vi "AlliGator All ROIs IRF Analysis.vi"(8 "error in (no error)":errorcluster, 11 "AlliGator Internal Variables DVR":refnum<data-value>) -> (0 "error out":errorcluster, 1 "# IRFs defined":i32, 2 "Message":string, 3 "AlliGator Internal Variables DVR":refnum<data-value>)   [LabVIEW 2021, in "AlliGator Decay Analysis.lvlib" / "AlliGator IRF.lvlib"]
doc: "Extracts the decays from all ROIs and stores them as IRFs for subsequent NLSF analysis."
uses:
  AlliGator IRF.lvlib
  AlliGator Internal Variables v2.ctl
  <vilib>/vision/Image Controls.llb/IMAQ Image.ctl
  AlliGator Gate Image Set.ctl
  AlliGator FLI Dataset Type.ctl
  AlliGator Data Series Type.ctl
  AlliGator Dataset Channel.ctl
  AlliGator Gate Arithmetic.ctl
  AlliGator Displayed Image.ctl
  Image/Named ROI Description.ctl
  AlliGator Decay Metadata v3.ctl
  AlliGator Decay Background Subtraction Info.ctl
  AlliGator Baseline Subtraction Method.ctl
  Graphs/XY Graph/XY Graph Plot Shift Parameters.ctl
  Graphs/XY Graph/XY Graph Plot Shift Method.ctl
  AlliGator Decay Extrapolation Parameters.ctl
  Phasor/Calibration Phasor (m, phi).ctl
  Phasor/Phasor Reference Series.ctl
  Phasor/Phasor Calibration Map v2.ctl
  Phasor/Phasor (g, s).ctl
  AlliGator Raw Phasor Plot Data v4.ctl
  Phasor/Phasor Standard Deviation Options.ctl
  AlliGator Phasor Multi-Harmonic Data.ctl
  Phasor/Phasor Harmonic Data.ctl
  AlliGator Decay Fit Options & Parameters v2.ctl
  Fits/IRF(X)PSED/Decay Fit Options v2.ctl
  Fits/Decay Convolution/Decay Model.ctl
  Fits/Residual Type.ctl
  Fits/IRF(X)PSED/Fit Weights Type.ctl
  Fits/Non-linear Fitting Method v2.ctl
  Fits/Fit Calculation Method.ctl
  Fits/Non-linear Fitting Algorithm.ctl
  AlliGator Decay Fit Parameter Constraints 2.ctl
  Fits/IRF(X)PSED/Decay Fit Parameters In List.ctl
  Fits/IRF(X)PSED/MLE Baseline Offset Type.ctl
  AlliGator Decay Preprocessing Parameters.ctl
  Fits/IRF(X)PSED/Decay Fit Parameters & Derived Quantities List.ctl
  AlliGator Variables List.ctl
  Variant/Variant to Data/Variant to U16.vi
  <vilib>/Utility/error.llb/Error Cluster From Error Code.vi
  AlliGator Abort.vi
  <vilib>/ErrorRing/Error Ring.xnode
  AlliGator Globals, Variables & Constants.lvlib
  Image/Image.lvlib
  AlliGator Decay Processing.lvlib
  AlliGator Source Image.lvlib
  Strings/Strings.lvlib
  Time/Time.lvlib
  AlliGator Decay Preprocessing.lvlib
  Notebook/Notebook.lvlib
  Rich Text Box/Rich Text Box.lvlib
  GUI/GUI.lvlib
  Variant/Variant to Data/Variant to Data.lvlib
  Phasor/Phasor.lvlib
  AlliGator Files.lvlib
  AlliGator Internal Variables.lvlib
  AlliGator Phasor Graph.lvlib
  Graphs/XY Graph/XY Graph Add-Ons.lvlib
  AlliGator Phasor Plot.lvlib
  Fits/Fits.lvlib
  AlliGator Decay Fit.lvlib
  AlliGator Decay Fit Parameter Map.lvlib
  AlliGator Settings.lvlib
  AlliGator Dual-Channel Datasets.lvlib
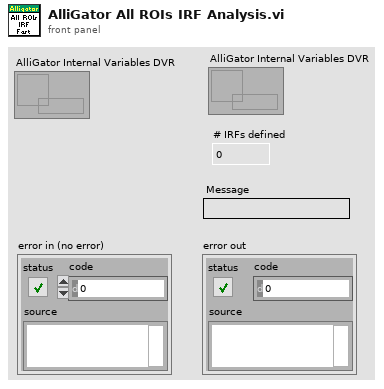
[diagram p1: front panel]
types:
  T1 = typedef "AlliGator Globals, Variables & Constants.lvlib/AlliGator Variables List.ctl" = enum16{"---- GUI ----", "Initialization Status", "State Indicators Refnum", "Original AlliGator Menu Items", "Current Action Loop State", "Script in progress", "Playback", "Loop Playback", "Search ROI Used", "Search ROI", "Decay Graph Max Legend Size", "Intensity Graph Max Legend Size", "Decay Statistics Graph Max Legend Size", "Phasor Graph Max Legend Size", "Phasor Ratio Graph Max Legend Size", "Lifetime Graph Max Legend Size", "---- Files ----", "Export Dataset Frames as Individual Files", "Show Batch Export Help Balloons", "Frames in Dataset", "ptu File Frame Start Indices", "Current Frame in Dataset", "Current Frame Timestamp", "------ Python Plugins ------", "Python Plugins Information", "Python Session", "Valid Python Session?", "---- Source Image ----", "Dataset Loaded", "Dataset Metadata", "Dataset Channel", "Dataset Data Description", "Background Dataset Metadata", "Background Dataset Channel", "Background Dataset Data Description", "Background File Subtraction", "Background File Path", "Background File Pile-up Correction", "Background File Pixel Well Capacity", "Background File Scaling Factor", "Source Image ROIs", "Current Source Image ROI", "Source Image ROI Event Refnum", "X_Source Image Display Range", "X_Source Image Palette Information", "Source Image Palette List", "Source Image Scale", "Current Dataset Load Settings", "Source Image:ROI Overlay Color", "---- Image Profile Window ----", "Image Profile:Overlay ROI in Source Image", "Image Profile Window Event Refnum", "Image Profile:IntensityType", "Image Profile:Intensity Average Type", "Image Profile:Intensity-weighted SDV", "Image Profile:Box Profile Type", "Image Profile Window Open", "Image Profile:Plotted Fit Parameter", "X_Type of Displayed Image", "X_Time Gate Slider", "Dataset Path", "Source Image Overlay to Erase", "Is Displayed Image Accumulated", "White Light Image Modified", "Mask Image Modified", "Macrotime Gate Separation", "------ Phasor Graph -------", "Phasor Graph:Show Line", "---- Phasor Plot ---", "Phasor Plot Parameters Changed", "FLI Dataset Modified since last Phasor Plot Calculation", "Phasor Harmonics Data", "Selected Phasor Harmonics", "Phasor Harmonic Manager Event Refnum", "Phasor Plot ROIs", "Current Phasor Plot ROI", "Phasor Plot ROI Event Refnum", "Phasor Plot Image Reference Points", "Phasor Plot Computed", "Phasor Plot Palette Information", "Phasor Plot Palette List", "Phasor Ratio Palette Information", "Phasor Ratio Palette List", "Phasor Image Scale", "Phasor Plot Image Overlay to Erase", "Phasor Plot Image Elements to Update", "Current Phasor Plot Calculation Parameters", "Current Phasor Calibration Options", "Reset Cumulated Phasor Plot", "Phasor Ratio Reference 1", "Phasor Ratio Lifetime Reference 1", "Phasor Ratio Reference 1 Frequency", "Phasor Ratio Reference 2", "Phasor Ratio Lifetime Reference 2", "Phasor Ratio Reference 2 Frequency", "---- Decay Analysis ----", "Number of Selected Decays to Fit", "LS Fit Results", "LAR Fit Results", "BS Fit Results", "Last Decay Max - Min", "Best Fit Parameters", "Best Fit Parameter Names", "Actual Size X", "Actual Size Y", "Binning X", "Binning Y", "Actual # Gates", "Dataset Number", "Gates to...", "Gates Skipped", "Gates to keep", "Gate Step", "Gate Separation", "Reversed Gates", "Pile-up Correction", "Pixel Well Capacity", "Background Subtracted", "Background Subtraction Method", "Background Definition Range", "Background File (deprecated)", "Number of Dataset Accumulated", "Array of Accumulated Dataset Paths", "Do Averaged Datasets", "Destination File Path", "Process Plot Target", "Use 1/D as Phasor Frequency", "---- Decay Fit Parameter Map -----", "Decay Fit Parameter Map Palette Information", "Decay Fit Parameter Map Palette List", "Local Decay Graph Window Event Refnum", "------- Local Decay Window ---------", "Use normalized IRF for convolution", "----- Miscellaneous ----", "Skippable Dialog Windows Status"}
  T2 = typedef "IMAQ Image.ctl" = refnum<image>
  T3 = typedef "Image.lvlib/Named ROI Description.ctl" = cluster{"ROI Descriptor":T4, "ROI Name":string, "Overlay Color":u32}
  T4 = typedef "ROI Descriptor" = cluster{"Global Rectangle":i32[], "Contours":cluster{"ID":enum32{"External", "Internal"}, "Type":u32, "Coordinates":i32[]}[]}
  T5 = typedef "AlliGator Internal Variables.lvlib/AlliGator Internal Variables v2.ctl" = cluster{"Displayed Image":T2, "White Light Image":T2, "Mask Image":T2, "ROI Mask Image":T2, "Current Dataset Images 1":T6, "Background Dataset Images 1":T6, "Current Dataset Images 2":T6, "Background Dataset Images 2":T6, "Current Dataset Arithmetic Images":T6, "Accumulated Dataset Images 1":T6, "Accumulated Dataset Images 2":T6, "Accumulated Dataset Arithmetic Images":T6, "Phasor Plot Image":T2, "Decay Fit Parameter Map Image":T2, "Single Data Point Path":path, "White Light Image Path":path, "Mask Image Path":path, "Time-Series Folder":path, "[Time-Series Paths]":path[], "Current Dataset":i32, "Single Dataset Type":T7, "Current Folder":string, "AlliGator Data Series Type":T8, "# Datasets":i32, "Dual-Channel Dataset":bool, "Selected Channel Name":string, "Dataset Channel":T9, "Channel Arithmetic":T10, "Dual-Channel Background Dataset":bool, "Background Channel":T9, "Dual-Channel Accumulated Dataset":bool, "Start Time":dbl, "[Time-Series Timestamps]":dbl[], "[Intensity Corrections]":dbl[], "Time Series Script":bool, "Type of Displayed Image":T11, "Gate Image Slide":u16, "# Gates":i32, "ROIs":T3[], "ROI Decay":cluster{"t Array":dbl[], "I Array":dbl[]}, "Valid Decay":bool, "Decay  Metadata":T12, "Reference Decay Plot Name":string, "Reference Decay":cluster{"t Array":dbl[], "I Array":dbl[]}, "Decay Shift Plot":cluster{"Time Stamps":dbl[], "Decay Shifts":dbl[]}, "[Decays Max Values]":sgl[], "[Decays Min Values]":sgl[], "Calibration Phasor":T18, "Calibration Phasor Series":T19, "Phasor Calibration Map":T20, "Calibration Map MD5 Digest":string, "Last Raw Phasor":T21, "Last Calibrated Phasor":T21, "Last Calibrated Phasor SDV":T21, "Phasor Graph:Phasor Plot":cluster{"g Array":dbl[], "s Array":dbl[]}, "Phasor Graph:Phasor SDV Plot":cluster{"g Array":dbl[], "s Array":dbl[]}, "[Phasor Graph:Raw Phasor Plots]":T22[], "Phasor Plot locked to Ref 1":i32, "[Phasor Plot(s) locked to Ref 1]":i32[], "[Phasor Plot(s) locked to Ref 2]":i32[], "[Pixel Phasors]":T21[], "[[Sum Image]]":dbl[][], "[[CSG Phasors]]":csg[][], "[[Valid Pixel?]]":bool[][], "I/m/phi Dataset":cluster{"I/m/phi Dataset?":bool, "Base Frequency":dbl[unit], "Harmonic Orders":u8[]}, "Multi Phasor Plot Data":T24, "Decay Fit Options & Parameters":T26, "Fit Options: Decay Preprocessing Parameters":T37, "Fit Options: Reference Decay":cluster{"t Array":dbl[], "I Array":dbl[]}, "Is Full Image Parameters Map":bool, "Is Single-Pixels Parameters Map":bool, "NLSF Parameters Map X Resolution":i32, "NLSF Parameters Map Y Resolution":i32, "[Single Decay Fit Parameters]":dbl[], "Fit Model":T28, "[[Multiple Decays Fit Parameters]]":dbl[][], "[[Multiple Decays Fit Parameter SDVs]]":dbl[][], "[[IRFs]]":dbl[][], "IRF Array Time Axis":dbl[], "Decay Array Time Axis":dbl[], "[Decay Fit Parameter Names]":T38[], "[[Phasor Ratios]]":dbl[][], "[[Average Lifetimes]]":dbl[][], "Amplitude Weighted Average Lifetime":bool, "[Decay Sum]":dbl[], "[[User-defined Quantities]]":dbl[][], "User-defined Quantity":string}
  T6 = typedef "AlliGator Files.lvlib/AlliGator Gate Image Set.ctl" = cluster{"SGL Image Max":T2, "SGL Image Sum":T2, "SGL Gate Images":T2[], "SGL Image Min":T2}
  T7 = typedef "AlliGator Files.lvlib/AlliGator FLI Dataset Type.ctl" = enum16{"HDF5 FLI Dataset", "Gate Image Folder", ".sdt FLI Dataset (Becker & Hickl)", ".ptu FLI Dataset (PicoQuant)", "SS1 FLI Dataset", "SS2 FLI Dataset", "I/m/phi Dataset", ".bin FLI Dataset (PicoQuant Binned)", ".bin FLI Dataset (Piccolo Binned)"}
  T8 = typedef "AlliGator Files.lvlib/AlliGator Data Series Type.ctl" = enum16{"Not a Supported Series", "Gate Images Folder Series", "SwissSPAD 2 Dataset Series", "B&H FLI Dataset Series", "PicoQuant PTU FLI Dataset Series", "PicoQuant BIN FLI Dataset Series", "Piccolo hist BIN FLI Dataset Series", "HDF5 FLI Dataset Series"}
  T9 = typedef "AlliGator Dual-Channel Datasets.lvlib/AlliGator Dataset Channel.ctl" = enum16{"G2", "INT"}
  T10 = typedef "AlliGator Settings.lvlib/AlliGator Gate Arithmetic.ctl" = enum16{"None", "INT-G2", "G2/INT*<INT>", "(1 - G2/INT)*<INT>"}
  T11 = typedef "AlliGator Source Image.lvlib/AlliGator Displayed Image.ctl" = enum16{"Single Gate", "Sum of All Gates", "Max of All Gates", "Min of All Gates", "-", "White Ligth Image", "Mask Image"}
  T12 = typedef "AlliGator Phasor Graph.lvlib/AlliGator Decay Metadata v3.ctl" = cluster{"ROI Descriptor":T4, "ROI Center":cluster{"X":i32, "Y":i32}, "Decay Background Subtraction Info":T13, "Decay Reverted":bool, "Decay Smoothened":bool, "Decay Straightened":bool, "Fitted Tau (Decay Straightening)":dbl, "Decay Shift Parameters":T15, "Decay Shifted":bool, "Decay Extrapolated":bool, "Decay Extrapolation Parameters":T17, "Decay Normalized":bool, "Fold Decay":bool, "# Folds":u32}
  T13 = typedef "AlliGator Decay Analysis.lvlib/AlliGator Decay Preprocessing.lvlib/AlliGator Decay Background Subtraction Info.ctl" = cluster{"Laser Period":dbl[unit], "Gate Duration":dbl[unit], "Baseline Subtraction Method":T14, "Background Definition Range":cluster{"Min Gate":dbl[unit], "Max Gate":dbl[unit]}, "Total Intensity w/o Bkgd Subtraction":dbl, "Bkgd-subtracted Intensity (exp)":dbl, "# Data Points":i32, "Background/Gate":dbl, "Fitted Lifetime":dbl[unit], "Bkgd-subtracted Intensity (theo)":dbl}
  T14 = typedef "AlliGator Decay Analysis.lvlib/AlliGator Decay Preprocessing.lvlib/AlliGator Baseline Subtraction Method.ctl" = enum16{"Mean", "Min", "Square Gated Single-Exponential", "File", "Constant"}
  T15 = typedef "XY Graph Add-Ons.lvlib/XY Graph Plot Shift Parameters.ctl" = cluster{"Type":T16, "Shift":dbl[unit], "Threshold":dbl, "Rotate":bool}
  T16 = typedef "XY Graph Add-Ons.lvlib/XY Graph Plot Shift Method.ctl" = enum16{"Default", "CFD", "Threshold", "Cross-Correlation"}
  T17 = typedef "AlliGator Decay Analysis.lvlib/AlliGator Decay Preprocessing.lvlib/AlliGator Decay Extrapolation Parameters.ctl" = cluster{"Additional Points":u32, "Head Fraction":dbl, "Fitted Tau":dbl, "Use Periodicity":bool, "Use Cursors":bool, "Tail Fraction":dbl}
  T18 = typedef "Phasor.lvlib/Calibration Phasor (m, phi).ctl" = cluster{"m":dbl, "phi":dbl, "Phasor Frequency":dbl[unit], "Reference Lifetime":dbl[unit]}
  T19 = typedef "Phasor.lvlib/Phasor Reference Series.ctl" = cluster{"m Array":dbl[], "phi Array":dbl[], "Phasor Frequency":dbl[unit], "Calibration Lifetime":dbl[unit]}
  T20 = typedef "Phasor.lvlib/Phasor Calibration Map v2.ctl" = cluster{"Phasor Frequency":dbl[unit], "Calibration Lifetime":dbl[unit], "ROI Centers":cluster{"X":i32, "Y":i32}[], "ROI Descriptors":T4[], "Map Resolution X":i32, "Map Resolution Y":i32, "z Array":cdb[]}
  T21 = typedef "Phasor.lvlib/Phasor (g, s).ctl" = cluster{"g":dbl, "s":dbl}
  T22 = typedef "AlliGator Phasor Graph.lvlib/AlliGator Raw Phasor Plot Data v4.ctl" = cluster{"Phasor Plot Name":string, "Raw Phasor Plot":T21[], "Phasor Frequency":dbl[unit], "[Decay Metadata]":T12[], "Raw Phasor Plot SDV":T21[], "Phasor SDV Options":T23, "[Calibration Phasor]":T18[]}
  T23 = typedef "Phasor.lvlib/Phasor Standard Deviation Options.ctl" = cluster{"Compute Estimated SDV":bool, "# Replicas":u32, "Use Estimated Average Phasor":bool}
  T24 = typedef "AlliGator Phasor Plot.lvlib/AlliGator Phasor Multi-Harmonic Data.ctl" = cluster{"Base Frequency":dbl[unit], "# Harmonics":u8, "Harmonic Orders":u8[], "Phasor Plot Settings Checksum":u64, "Phasor Harmonic Data Array":T25[]}
  T25 = typedef "Phasor.lvlib/Phasor Harmonic Data.ctl" = cluster{"Phasor Harmonic Name":string, "Phasor Plot Settings Checksum":u64, "Phasor Frequency":dbl[unit], "Base Frequency":dbl[unit], "Harmonic Order":u8, "Phasor Plot Parameters":string, "Phasor Array [[CSG]]":csg[][], "Dataset File Path":path}
  T26 = typedef "AlliGator Decay Fit Parameter Map.lvlib/AlliGator Decay Fit Options & Parameters v2.ctl" = cluster{"SYNC Period":dbl[unit], "Fit Options":T27, "Fit Parameter Constraints":T34[], "MLE Baseline Offset":dbl, "MLE Baseline Offset Type":T36}
  T27 = typedef "Fits.lvlib/Decay Fit Options v2.ctl" = cluster{"Show Fit Residuals":bool, "Fit Model":T28, "Residual Type":T29, "Max Decay Percentile":dbl, "Min Decay Percentile":dbl, "Show Full Decay":bool, "Weights":T30, "Fitting Method":T31, "Compute Parameter Uncertainties":bool, "Periodic Boundaries":bool, "Model Calculation":T32, "Period":dbl[unit], "Termination Criteria":cluster{"Max Iterations":i32, "Max Function Calls":i32, "Max Time":dbl[unit], "Function Tolerance":dbl, "Parameter Tolerance":dbl, "Gradient Tolerance":dbl, "Min Lambda":dbl, "Max Lambda":dbl, "Initial Tick Count":u32}, "Offset Resolution":dbl[unit], "Use Local IRF":bool, "Fitting Algorithm":T33}
  T28 = typedef "Fits.lvlib/Decay Model.ctl" = enum16{"1-Exponential", "2-Exponentials"}
  T29 = typedef "Fits.lvlib/Residual Type.ctl" = enum16{"Standard", "Normalized", "Reduced"}
  T30 = typedef "Fits.lvlib/Fit Weights Type.ctl" = enum16{"Unweighted", "1/Variance", "Best of All"}
  T31 = typedef "Fits.lvlib/Non-linear Fitting Method v2.ctl" = enum16{"Least Square", "Least Absolute Residual", "Bisquare", "MLE", "-", "Best of All"}
  T32 = typedef "Fits.lvlib/Fit Calculation Method.ctl" = enum16{"Simulation", "Convolution", "Integration"}
  T33 = typedef "Fits.lvlib/Non-linear Fitting Algorithm.ctl" = enum16{"Levenberg-Marquardt", "Trust-Region Dogleg"}
  T34 = typedef "AlliGator Decay Analysis.lvlib/AlliGator Decay Fit.lvlib/AlliGator Decay Fit Parameter Constraints 2.ctl" = cluster{"Fit Parameter":T35, "Min Value":dbl, "Max Value":dbl, "Global":bool, "Used":bool}
  T35 = typedef "Fits.lvlib/Decay Fit Parameters In List.ctl" = enum16{"Offset", "Baseline", "A_1", "tau_1", "A_2", "tau_2"}
  T36 = typedef "Fits.lvlib/MLE Baseline Offset Type.ctl" = enum32{"Absolute", "Percentage"}
  T37 = typedef "AlliGator Decay Analysis.lvlib/AlliGator Decay Preprocessing.lvlib/AlliGator Decay Preprocessing Parameters.ctl" = cluster{"Background Subtraction":bool, "Straighten Decay":bool, "Reverse Gates":bool, "1-Normalized Decay":bool, "Smoothen Decay":bool, "Smoothing Parameter":dbl, "Shift Decay":bool, "Decay Shift Parameters":T15, "Extrapolate Decay":bool, "Additional Points":u32, "Head Fraction":dbl, "Pixel-Normalize Decay":bool, "Use Periodicity":bool, "Use Cursors":bool, "Tail Fraction":dbl, "Use Decay Pre-Processing":bool, "Fold Decay":bool, "# Folds":u32, "[0-1]-Normalized Decay":bool}
  T38 = typedef "Fits.lvlib/Decay Fit Parameters & Derived Quantities List.ctl" = enum16{"Offset", "Baseline", "A_1", "tau_1", "A_2", "tau_2", "<tau>_a", "f1_a", "f2_a", "<tau>_i", "f1_i", "f2_i", "-", "R^2", "Chi^2"}
  T39 = typedef "AlliGator Settings.lvlib/AlliGator Pixel Counts Constraints.ctl" = cluster{"High Count Pixels Rejection Options":T40, "Low Count Pixels Rejection Options":T41}
  T40 = typedef "AlliGator Settings.lvlib/AlliGator High Count Pixels Rejection Options.ctl" = cluster{"Background High Threshold Factor":dbl, "Fixed High Background Threshold":dbl, "Reject High Count Pixels":bool, "High Percentile":dbl}
  T41 = typedef "AlliGator Settings.lvlib/AlliGator Low Count Pixels Rejection Options.ctl" = cluster{"Background Low Threshold Factor":dbl, "Fixed Low Background Threshold":dbl, "Reject Low Count Pixels":bool, "Low Percentile":dbl}
  T42 = cluster{"Decay Peak Constraint":bool, "Min":dbl, "Max":dbl}
  T43 = typedef "Rich Text Box.lvlib/Text Formatting.ctl" = cluster{"Font":string, "Text Color":T44, "Text Background Color":T44, "Text Style":enum16{"Regular", "Bold", "Italic", "Underline", "Strikeout"}, "Font Size (Points)":dbl, "Text Alignment":i32}
  T44 = typedef "Rich Text Box.lvlib/Text Colors.ctl" = enum16{"Unchanged", "Black", "Blue", "Brown", "Gray", "Green", "Orange", "Pink", "Red", "White"}
  T45 = cluster{"t Axis":dbl[], "ROI Intensity Array":dbl[]}
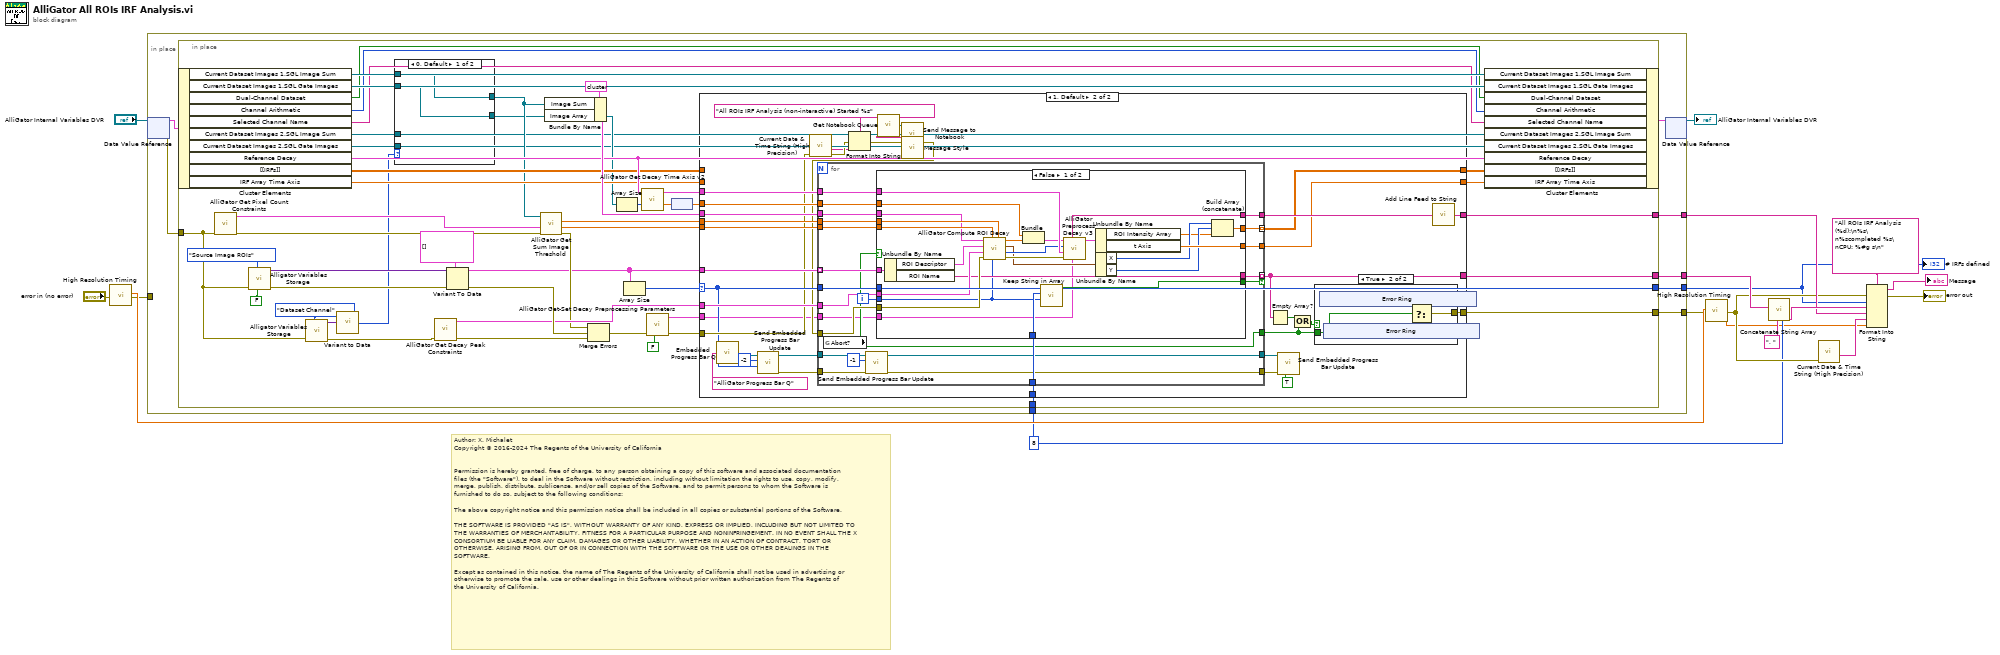
[diagram p0: block diagram]
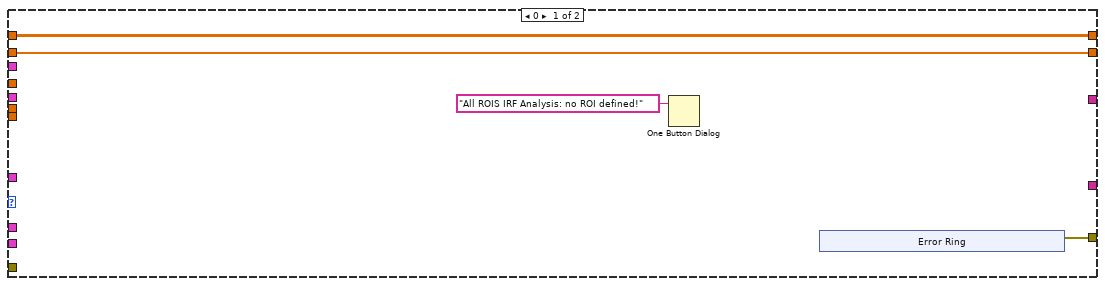
[diagram p3: hidden frame]
diagram:
  w6 = 8 ("Max Number of Elements (None: -1)")
  # "Author: X. Michalet\nCopyright © 2016-2024 The Regents of the University of California\n \n\nPermission is hereby granted, free of charge, to any person obtaining a copy of this software and associated documentation files (the \"Software\"), to deal in the Software without restriction, including without limitation the rights to use, copy, modify, merge, publish, distribute, sublicense, and/or sell copies of the Software, and to permit persons to whom the Software is furnished to do so, subject to the following conditions:\n\nThe above copyright notice and this permission notice shall be included in all copies or substantial portions of the Software.\n\nTHE SOFTWARE IS PROVIDED \"AS IS\", WITHOUT WARRANTY OF ANY KIND, EXPRESS OR IMPLIED, INCLUDING BUT NOT LIMITED TO THE WARRANTIES OF MERCHANTABILITY, FITNESS FOR A PARTICULAR PURPOSE AND NONINFRINGEMENT. IN NO EVENT SHALL THE X CONSORTIUM BE LIABLE FOR ANY CLAIM, DAMAGES OR OTHER LIABILITY, WHETHER IN AN ACTION OF CONTRACT, TORT OR OTHERWISE, ARISING FROM, OUT OF OR IN CONNECTION WITH THE SOFTWARE OR THE USE OR OTHER DEALINGS IN THE SOFTWARE.\n\nExcept as contained in this notice, the name of The Regents of the University of California shall not be used in advertising or otherwise to promote the sale, use or other dealings in this Software without prior written authorization from The Regents of the University of California."
  n1 = call "High Resolution Timing.vi"("Error In"="error in (no error)") -> ("elapsed (relative) seconds"=w13:dbl, "Error Out"=w10:errorcluster)  [unwired: 16 in, 1 out]
  n2 = in-place {
    in-place-border: [w24] -> w7
    in-place-border: [w23] -> w11
    in-place-border: w10 -> [_]
    in-place-border: [w21] -> w9
    in-place-border: [w20] -> w5
    in-place-border: w6 -> [w19]
    n3 = in-place-dvr #1("AlliGator Internal Variables DVR") -> (w26:T5, w22:errorcluster)
    n4 = in-place {
      in-place-border: w22 -> [w29]
      in-place-border: [w57] -> w24
      in-place-border: [w48] -> w23
      in-place-border: [w56] -> w21
      in-place-border: [w50] -> w20
      in-place-border: w19 -> [w49]
      n5 = in-place-cluster #2(w26) -> ("Current Dataset Images 1.SGL Image Sum"=w38:T2, "Current Dataset Images 1.SGL Gate Images"=w37:T2[], "Dual-Channel Dataset"=w32:bool, "Channel Arithmetic"=w33:T10, "Selected Channel Name"=w34:string, "Current Dataset Images 2.SGL Image Sum"=w36:T2, "Current Dataset Images 2.SGL Gate Images"=w35:T2[], "Reference Decay"=w58:cluster{"t Array":dbl[], "I Array":dbl[]}, "[[IRFs]]"=w45:dbl[][], "IRF Array Time Axis"=w44:dbl[])
      n6 = call "AlliGator Get Pixel Count Constraints.vi"("error in (no error)"=w29) -> ("error out"=w67:errorcluster, "Pixel Count Constraints"=w68:T39)  [unwired: 9 in]
      n7 = call "Alligator Variables Storage.vi"("Get(F)/Set"=FALSE, "AlliGator Variable"=AlliGator_Variables_List."Source Image ROIs" ("Alligator Variable"), "Error In"=w29) -> ("Error Out"=w71:errorcluster, "Data out"=w72:variant)  [unwired: 6 in, 1 out]
      n8 = call "Alligator Variables Storage.vi"("AlliGator Variable"=AlliGator_Variables_List."Dataset Channel" ("Alligator Variable"), "Error In"=w29) -> ("Error Out"=w28:errorcluster, "Data out"=w30:variant)  [unwired: 7 in, 1 out]
      n9 = call-poly "Variant to Data.vi"("Variant"=w30) -> ("U16 Value"=w27:u16)  [unwired: 8 in]
      n10 = case shown="0, Default" w27 {
        tunnel: [w75 w77] -> w40
        tunnel: w36 -> [_ w77]
        tunnel: [w74 w76] -> w39
        tunnel: w35 -> [_ w76]
        tunnel: w38 -> [w75 _]
        tunnel: w37 -> [w74 _]
        frame 0, Default {
        }
        frame 1 {
        }
      }
      n11 = call "AlliGator Get Decay Peak Constraints.vi"("error in (no error)"=w28) -> ("Error Out"=w63:errorcluster, "Decay Peak Constraints"=w62:T42)  [unwired: 9 in]
      n12 = Variant To Data(error in=w71, type=T3[] [] ("Stored ROIs in"), Variant=w72) -> (data=w51:T3[], error out=w66:errorcluster)
      n13 = call "AlliGator Get Sum Image Threshold.vi"("error in (no error)"=w67, "Pixel Counts Constraints"=w68, "Image in"=w40) -> ("error out"=w55:errorcluster, "Pixel Threshold Low"=w64:sgl, "Pixel Threshold High"=w65:sgl)  [unwired: 2 in, 4 out]
      n14 = Bundle By Name(cluster=cluster{"Image Sum":T2, "Image Array":T2[]} {"Image Sum"=refnum, "Image Array"=[]} ("Images"), "Image Sum"=w40, "Image Array"=w39) -> (w61:cluster{"Image Sum":T2, "Image Array":T2[]})
      n15 = Merge Errors(w55, w66, w63) -> (w47:errorcluster)
      n16 = Array Size(array=w39) -> (size(s)=w60:i32)
      n17 = Array Size(array=w51) -> (size(s)=w50:i32)
      n18 = call "AlliGator Get Decay Time Axis v2.vi"("Number of Gates"=w60) -> ("t Array"=w59:dbl[unit][])  [unwired: 14 in]
      n19 = call "AlliGator Get-Set Decay Preprocessing Parameters.vi"("Get (F)/Set"=FALSE, "Error In"=w47) -> ("Error Out"=w46:errorcluster, "Decay Preprocessing Parameters out"=w42:T37)  [unwired: 8 in]
      n20 = node(w59) -> (w54:dbl[])
      n21 = case shown="1, Default" w50 {
        selector: w50 -> [_ w92]
        tunnel: w65 -> [_ w121]
        tunnel: w64 -> [_ w120]
        tunnel: w62 -> [_ w119]
        tunnel: w61 -> [_ w118]
        tunnel: w58 -> [_ w117]
        tunnel: [w79 w116] -> w57
        tunnel: [_ w112] -> w56
        tunnel: w54 -> [_ w111]
        tunnel: [w80 w109] -> w53
        tunnel: [w81 w108] -> w52
        tunnel: w51 -> [_ w107]
        tunnel: w49 -> [_ w106]
        tunnel: [_ w105] -> w48
        tunnel: w46 -> [_ w98]
        tunnel: w45 -> [w81 _]
        tunnel: w44 -> [w80 _]
        tunnel: w42 -> [_ w87]
        frame 0 {
          n22 = One Button Dialog(message="All ROIS IRF Analysis: no ROI defined!") -> ()  [unwired: 1 in, 1 out]
          n23 = xnode "Error Ring"() -> ("error out"=w79:errorcluster)
        }
        frame 1, Default {
          n24 = call "Embedded Progress Bar Q.vi"("Progress Bar Queue Name"="AlliGator Progress Bar Q") -> ("Progress Bar Queue"=w95:refnum<queue>)  [unwired: 6 in]
          n25 = call "Send Embedded Progress Bar Update.vi"("Max Iterations N"=w92, "Current Iteration i (i or -1: standard or || iteration; 0 or -2: first standard or || iteration)"=-2 ("Current Iteration i (-1: || iteration, -2: first || iteration)"), "Progress Bar Queue in"=w95) -> ("Error Out"=w91:errorcluster, "Progress Bar Queue out"=w93:refnum<queue>)  [unwired: 7 in]
          n26 = call "Current Date & Time String (High Precision).vi"("Error In"=w98) -> ("Error Out"=w100:errorcluster, "on <Date> at <Time>"=w86:string)  [unwired: 7 in, 2 out]
          n27 = Format Into String(format string="All ROIs IRF Analysis (non-interactive) Started %s", error in=w100, w86) -> (resulting string=w97:string, error out=w102:errorcluster)  [unwired: 1 in]
          n28 = call "Get Notebook Queue.vi"() -> ("Notebook Queue"=w101:refnum<queue>)  [unwired: 9 in]
          n29 = call "Message Style.vi"() -> ("Message Formatting"=w103:T43)
          n30 = call "Send Message to Notebook.vi"("Text Formatting"=w103, "Error In"=w102, "Message"=w97, "Notebook Queue"=w101) -> ("Error Out"=w99:errorcluster)  [unwired: 4 in, 1 out]
          n31 = for {
            tunnel: w107 -> [w156] mode=indexing
            tunnel: w121 -> [w155]
            tunnel: w120 -> [w154]
            tunnel: w118 -> [w153]
            tunnel: w119 -> [w152]
            tunnel: [w140] -> w110
            tunnel: w111 -> [w148]
            tunnel: w117 -> [w149]
            tunnel: [w150] -> w105 mode=indexing if=w144
            tunnel: w99 -> [w151]
            tunnel: [w147] -> w113
            tunnel: [w146] -> w109
            tunnel: [w145] -> w108 mode=indexing
            tunnel: w92 -> [w142]
            tunnel: w106 -> [w141]
            tunnel: w93 -> [w138]
            tunnel: w91 -> [w137]
            tunnel: [w136] -> w90
            tunnel: [w135] -> w89
            tunnel: w87 -> [w134]
            i -> [w143]
            n32 = global read "AlliGator Abort.vi" "Abort?"() -> (w140:bool)
            n33 = call "Send Embedded Progress Bar Update.vi"("Error In"=w137, "Current Iteration i (i or -1: standard or || iteration; 0 or -2: first standard or || iteration)"=-1 ("Current Iteration i (-1: || iteration, -2: first || iteration)"), "Progress Bar Queue in"=w138) -> ("Error Out"=w135:errorcluster, "Progress Bar Queue out"=w136:refnum<queue>)  [unwired: 7 in]
            n34 = case shown="False" w140 {
              tunnel: w156 -> [w183 _]
              tunnel: w155 -> [w182 _]
              tunnel: w154 -> [w181 _]
              tunnel: w153 -> [w180 _]
              tunnel: w152 -> [w179 _]
              tunnel: w151 -> [w178 _]
              tunnel: [w177 _] -> w150
              tunnel: w149 -> [w175 _]
              tunnel: w148 -> [w173 _]
              tunnel: [w170 _] -> w147
              tunnel: [w166 _] -> w146
              tunnel: [w162 _] -> w145
              tunnel: [w161 _] -> w144
              tunnel: w143 -> [w157 _]
              tunnel: w142 -> [w160 _]
              tunnel: w141 -> [w159 _]
              tunnel: w134 -> [w158 _]
              frame False {
                n35 = Unbundle By Name(w183) -> ("ROI Descriptor"=w176:T4, "ROI Name"=w177:string)
                n36 = call "AlliGator Compute ROI Decay.vi"("Pixel Threshold High"=w182, "Loop ID"=w157, "Pixel Threshold Low"=w181, "error in (no error)"=w178, "Decay Peak  Constraints"=w179, "ROI Descriptor"=w176, "Images"=w180) -> ("error out"=w174:errorcluster, "# Valid Pixels"=w169:i32, "ROI Center"=w167:cluster{"X":i32, "Y":i32}, "Decay Points"=w172:dbl[])  [unwired: 1 out]
                n37 = Bundle(w173, "Decay Points"=w172) -> (w171:cluster{dbl[], "Decay Points":dbl[]})  [unwired: 1 in]
                n38 = call "Keep String in Array.vi"("Current Index"=w157, "Max Number of Strings (8)"=w159, "Number of Elements"=w160) -> ("Keep String"=w161:bool)  [unwired: 8 in]
                n39 = call "AlliGator Preprocess Decay v3.vi"("Decay Preprocessing Parameters"=w158, "Error In"=w174, "Time-Gated Reference Decay"=w175, "# Pixels"=w169, "Decay (in)"=w171) -> ("Decay (out)"=w168:T45, "Message"=w170:string)  [unwired: 3 in, 2 out]
                n40 = Unbundle By Name(w168) -> ("ROI Intensity Array"=w163:dbl[], "t Axis"=w166:dbl[])
                n41 = Unbundle By Name(w167) -> ("X"=w165:i32, "Y"=w164:i32)
                n42 = Build Array (concatenate)(w165, w164, w163) -> (w162:dbl[])
              }
              frame True {
              }
            }
          }
          n43 = Empty Array?(array=w105) -> (empty?=w114:bool)
          n44 = call "Send Embedded Progress Bar Update.vi"("Stop Progress Bar (F)"=TRUE, "Error In"=w89, "Progress Bar Queue in"=w90) -> ()  [unwired: 7 in, 2 out]
          n45 = Compound Arithmetic op=OR(w114, w110) -> (w115:bool)
          n46 = case shown="True" w115 {
            tunnel: [_ w123] -> w116
            tunnel: w110 -> [_ w125]
            frame False {
            }
            frame True {
              n47 = xnode "Error Ring"() -> ("error out"=w124:errorcluster)
              n48 = xnode "Error Ring"() -> ("error out"=w122:errorcluster)
              n49 = Select(t=w124, s=w125, f=w122) -> (s? t:f=w123:errorcluster)
            }
          }
          n50 = call "Add Line Feed to String.vi"("String"=w113) -> ("String\\n"=w112:string)  [unwired: 8 in]
        }
      }
      n51 = in-place-cluster #2("Current Dataset Images 1.SGL Image Sum"=w38, "Current Dataset Images 1.SGL Gate Images"=w37, "Dual-Channel Dataset"=w32, "Channel Arithmetic"=w33, "Selected Channel Name"=w34, "Current Dataset Images 2.SGL Image Sum"=w36, "Current Dataset Images 2.SGL Gate Images"=w35, "Reference Decay"=w58, "[[IRFs]]"=w52, "IRF Array Time Axis"=w53) -> (w25:T5)
    }
    n52 = in-place-dvr #1(w25) -> (→"AlliGator Internal Variables DVR":refnum<data-value>)  [unwired: 1 out]
  }
  "# IRFs defined" <- w5
  n53 = call "High Resolution Timing.vi"("relative seconds (NaN)"=w13, "Error In"=w7) -> ("elapsed (relative) seconds"=w2:dbl, "Error Out"=w8:errorcluster)  [unwired: 15 in, 1 out]
  n54 = call "Concatenate String Array.vi"("Max Number of Elements (None: -1)"=w6, "Separator (TAB)"=", ", "String Array"=w11) -> ("Formatted String"=w12:string)  [unwired: 8 in]
  n55 = call "Current Date & Time String (High Precision).vi"("Error In"=w8) -> ("on <Date> at <Time>"=w3:string)  [unwired: 7 in, 3 out]
  n56 = Format Into String(format string="All ROIs IRF Analysis (%d):\n%s\n%scompleted %s\nCPU: %#g s\n", error in=w8, w5, w12, w9, w3, w2) -> (resulting string=→"Message":string, error out=→"error out":errorcluster)  [unwired: 1 in]
